vi "LimitSwitchWrap.vi"(8 "error in":errorcluster, 11 "DigitalInputDevRef":T1) -> (0 "error out":errorcluster, 2 "Triggered":bool, 3 "DigitalInputDevRef 2":T1)   [LabVIEW 2013]
uses:
  <vilib>/Rock Robotics/WPI/DigitalInput/WPI_DigitalInputDevRef.ctl
  <vilib>/Rock Robotics/SystemInterfaces/DIO/FPGA_DIOChannel.ctl
  <vilib>/Rock Robotics/SystemInterfaces/Typedef/FPGA_TypedefDigitalModule.ctl
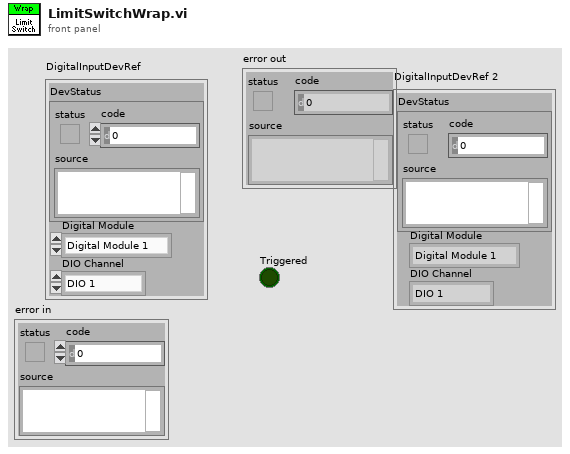
[diagram p1: front panel]
types:
  T1 = typedef "WPI_DigitalInputDevRef.ctl" = cluster{"DevStatus":errorcluster, "DIO Channel":T2, "Digital Module":T3}
  T2 = typedef "FPGA_DIOChannel.ctl" = enum8{"DIO 1", "DIO 2", "DIO 3", "DIO 4", "DIO 5", "DIO 6", "DIO 7", "DIO 8", "DIO 9", "DIO 10", "DIO 11", "DIO 12", "DIO 13", "DIO 14", "Invalid"}
  T3 = typedef "FPGA_TypedefDigitalModule.ctl" = enum16{"Digital Module 1", "Digital Module 2"}
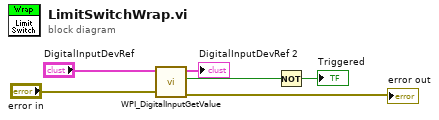
[diagram p0: block diagram]
diagram:
  n1 = call <vilib>:"WPI_DigitalInputGetValue.vi"("error in (no error)"="error in", "DigitalInputDevRef"="DigitalInputDevRef") -> ("error out"=→"error out":errorcluster, "Value"=w6:bool, "DigitalInputDevRef"=→"DigitalInputDevRef 2":T1)  [unwired: 7 in]
  n2 = Not(x=w6) -> (.not. x?=→"Triggered":bool)
